vi "Simulate Analog Sensor.vi"() -> ()   [LabVIEW 2020]
uses:
  Control/State - eFGV.ctl
panel:
  in  "Reset":bool
  in  "AI3":dbl(slide) scale=0.0..20000.0
  in  "AI2":dbl(slide) scale=0.0..20000.0
  in  "AI1":dbl(slide) scale=0.0..20000.0
  in  "AI0":dbl(slide) scale=0.0..20000.0
  in  "stop":bool
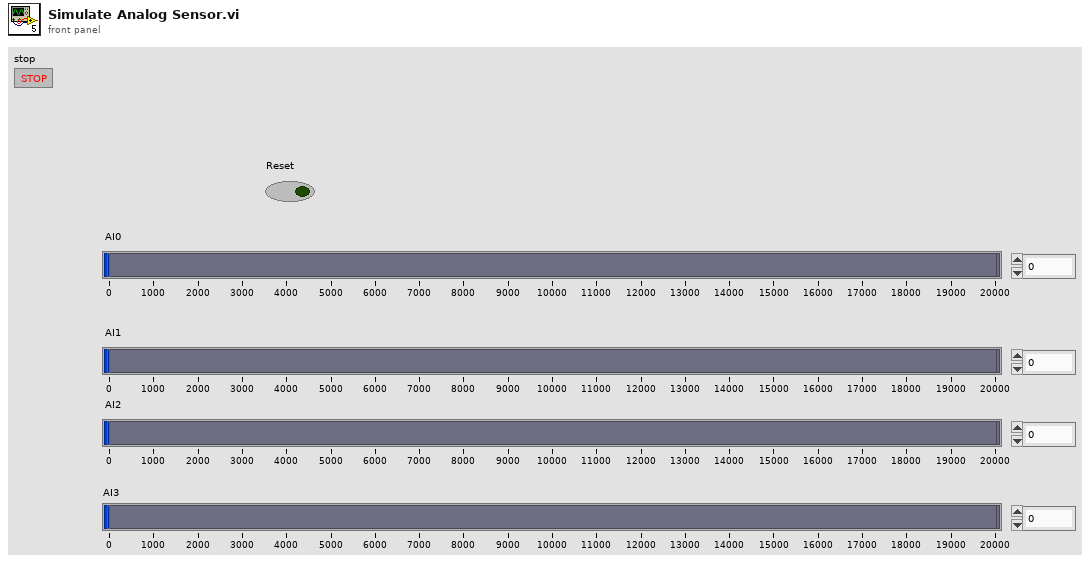
[diagram p1: front panel]
types:
  T1 = typedef "State - eFGV.ctl" = enum16{"Init", "Read", "Write", "Exit"}
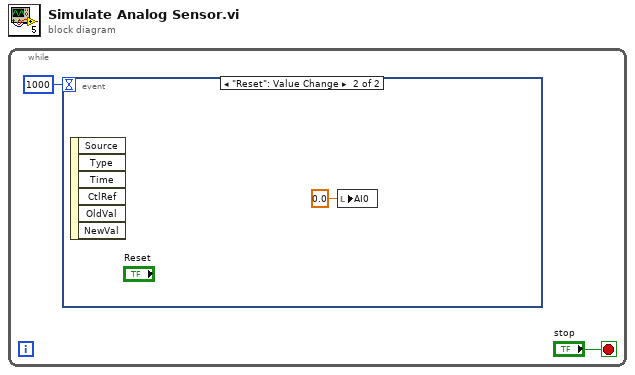
[diagram p0: block diagram]
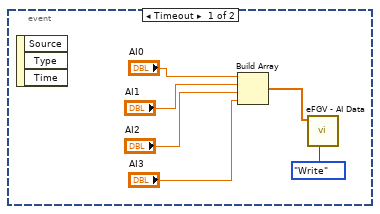
[diagram p2: hidden frame]
diagram:
  n1 = while {
    stop <- "stop" stop-if-true
    n2 = event shown="[1] \"Reset\": Value Change" {
      selector: _ -> [_ _]
      dyn-events: _ -> [_ _]
      timeout: 1000 -> [_ _]
      event Timeout {
        n3 = event-data() -> ()  [unwired: 1 in, 3 out]
        n4 = Build Array("AI0", "AI1", "AI2", "AI3") -> (w3:dbl[])
        n5 = call "eFGV - AI Data.vi"("States"=State_-_eFGV."Write", "Event AI Data"=w3) -> ()  [unwired: 8 in, 2 out]
      }
      event "Reset": Value Change {
        n6 = event-data() -> ()  [unwired: 1 in, 6 out]
        n7 = local write "AI0"(0.0 ("AI0")) -> ()
      }
    }
  }
